vi "Get GPS Data.vi"(8 "error in (no error)":errorcluster, 10 "sensor data":string, 11 "previous partial sentence":string) -> (0 "error out":errorcluster, 2 "GPS data":T1 {"oldest read timestamp" format="%^<%.3X\n%x>T"}, 3 "remaining partial sentence":string)   [LabVIEW 2017, in "NMEA API.lvlib"]
doc: "Parses <B>sensor data</B> in the NMEA format from GPS receivers and returns common <B>GPS data</B>, such as the latitude and longitude of a reading."
uses:
  <vilib>/robotics/Protocols/NMEA/NMEA API.lvlib
  <vilib>/robotics/Protocols/NMEA/Advanced/Instrument Specific Poly VIs/GPS/Parse GLL Sentence.vi
  <vilib>/robotics/Protocols/NMEA/Advanced/Instrument Specific Poly VIs/GPS/Parse GGA Sentence.vi
  <vilib>/robotics/Protocols/NMEA/Advanced/Instrument Specific Poly VIs/GPS/Parse RMC Sentence.vi
  <vilib>/robotics/Utilities/NI_Robotics Utilities.lvlib
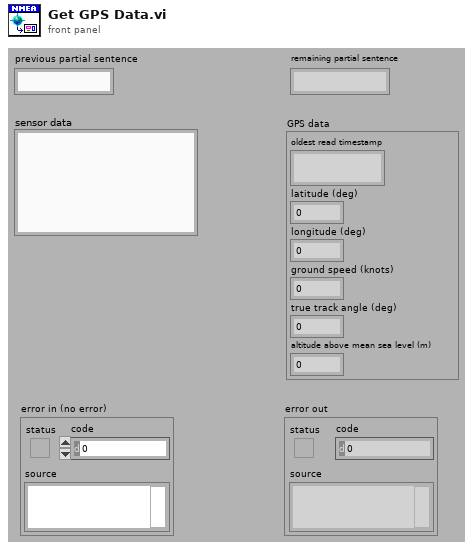
[diagram p1: front panel]
types:
  T1 = cluster{"oldest read timestamp":timestamp, "latitude (deg)":dbl, "longitude (deg)":dbl, "ground speed (knots)":dbl, "true track angle (deg)":dbl, "altitude above mean sea level (m)":dbl}
  T2 = cluster{"oldest read timestamp":timestamp, "latitude":dbl, "longitude":dbl, "speed over ground (knots)":dbl, "true track angle (deg)":dbl, "altitude above mean sea level":dbl}
  T3 = cluster{"Oldest Read Timestamp":timestamp, "Latitude":dbl, "Longitude":dbl, "Speed over Ground (Knots)":dbl, "True Track Angle (Deg)":dbl, "Altitude Above Mean Sea Level":dbl}
  T4 = typedef "NMEA API.lvlib/RMC Data.ctl" = cluster{"time of fix":cluster{"included?":bool, "time (UTC)":timestamp}, "status":cluster{"included?":bool, "value":u16}, "latitude":cluster{"included?":bool, "latitude (deg)":dbl}, "longitude":cluster{"included?":bool, "longitude (deg)":dbl}, "ground speed":cluster{"included?":bool, "speed (knots)":dbl}, "true track angle":cluster{"included?":bool, "angle (deg)":dbl}, "magnetic variation":cluster{"included?":bool, "variation (deg)":dbl}, "type of fix":cluster{"included?":bool, "mode":u16}}
  T5 = typedef "NMEA API.lvlib/GGA Data.ctl" = cluster{"time of fix":cluster{"included?":bool, "time (UTC)":timestamp}, "latitude":cluster{"included?":bool, "latitude (deg)":dbl}, "longitude":cluster{"included?":bool, "longitude (deg)":dbl}, "fix quality":cluster{"included?":bool, "quality":u16}, "number of satellites in view":cluster{"included?":bool, "number of satellites":i8}, "horizontal dilution of precision":cluster{"included?":bool, "horizontal DOP":dbl}, "altitude above mean sea level":cluster{"included?":bool, "altitude (m)":dbl}, "height of geoid above WGS84":cluster{"included?":bool, "height of geoid (m)":dbl}, "time since last DGPS update":cluster{"included?":bool, "time (s)":dbl}, "DGPS station ID number":cluster{"included?":bool, "station ID number":dbl}}
  T6 = typedef "NMEA API.lvlib/GLL Data.ctl" = cluster{"latitude":cluster{"included?":bool, "latitude (deg)":dbl}, "longitude":cluster{"included?":bool, "longitude (deg)":dbl}, "time of fix":cluster{"included?":bool, "time (UTC)":timestamp}, "status":cluster{"included?":bool, "value":u16}, "type of fix":cluster{"included?":bool, "mode":u16}}
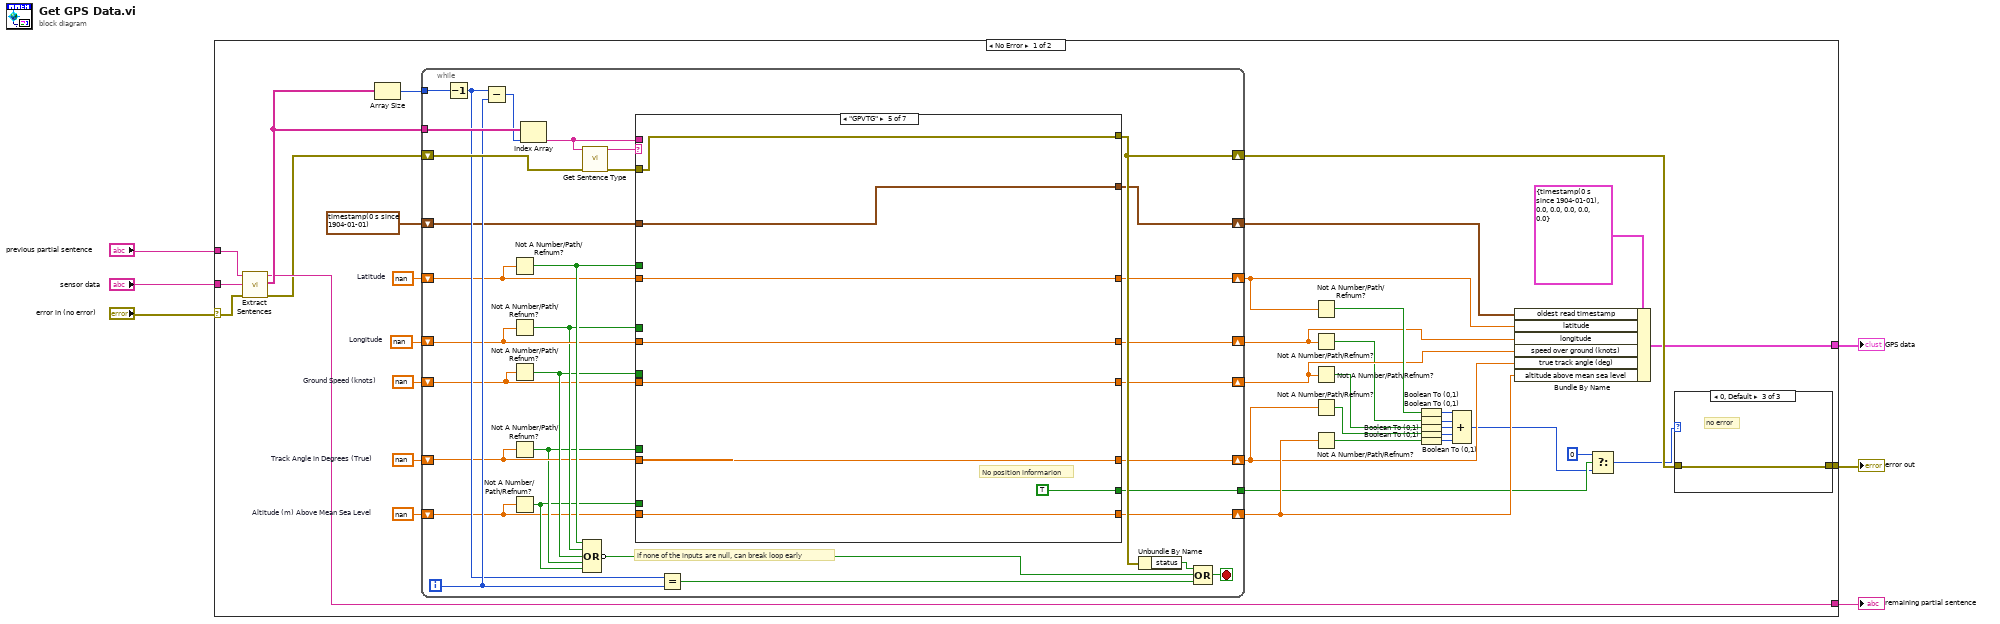
[diagram p0: block diagram]
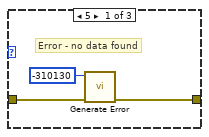
[diagram p2: hidden frame]
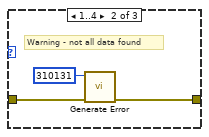
[diagram p3: hidden frame]
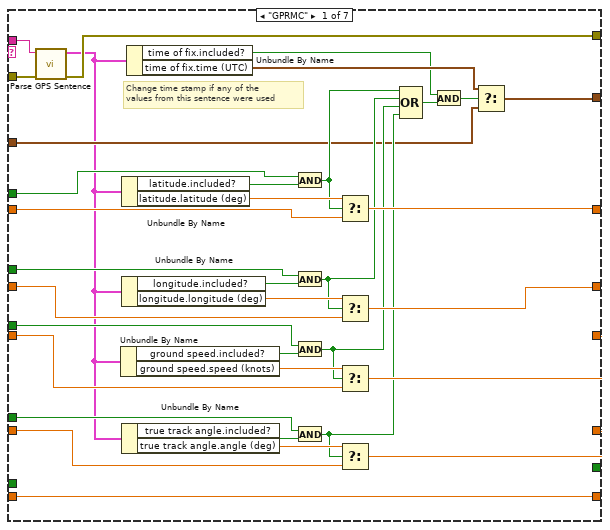
[diagram p4: hidden frame]
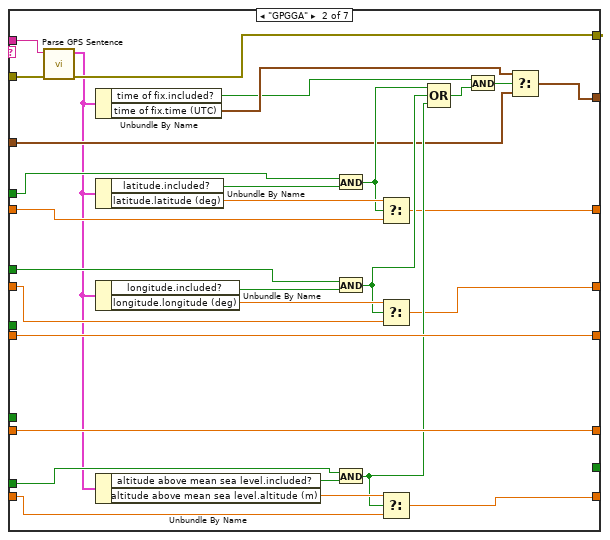
[diagram p5: hidden frame]
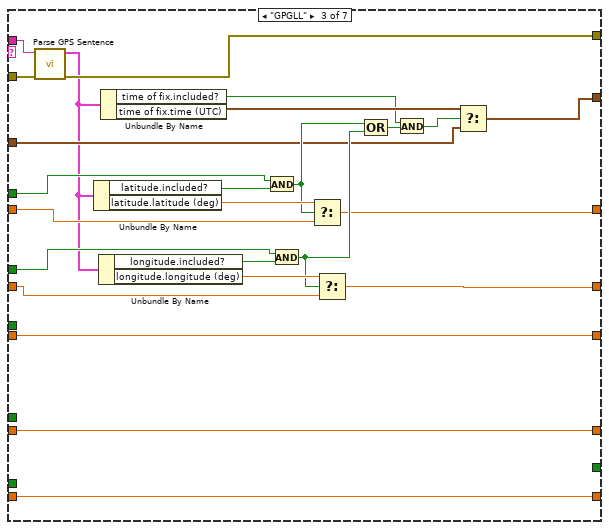
[diagram p6: hidden frame]
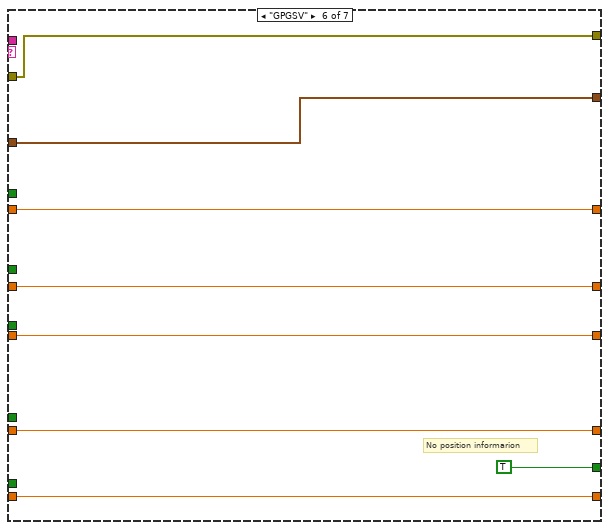
[diagram p8: hidden frame]
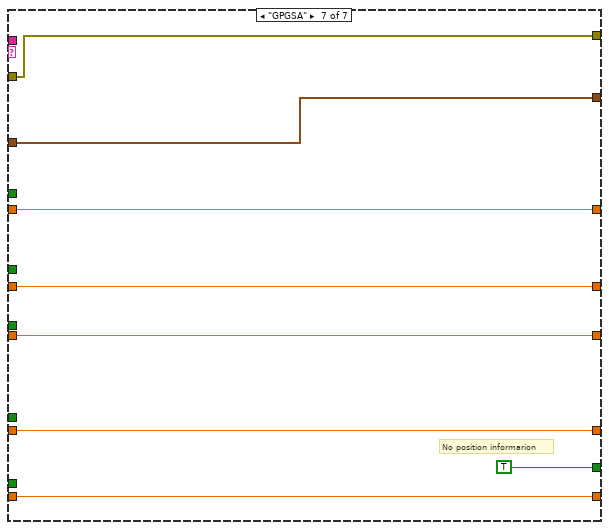
[diagram p9: hidden frame]
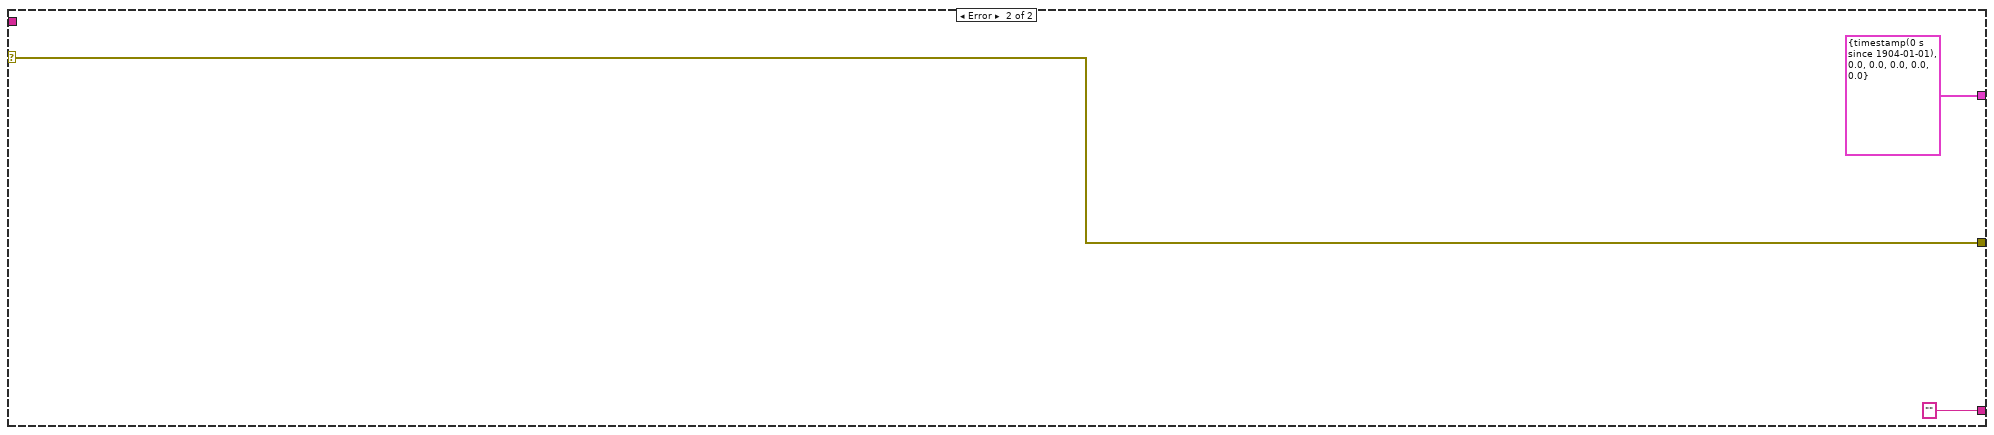
[diagram p10: hidden frame]
diagram:
  n1 = case shown="No Error" "error in (no error)" {
    selector: "error in (no error)" -> [w21 w206]
    tunnel: [w41 w206] -> w5
    tunnel: "sensor data" -> [w30 _]
    tunnel: "previous partial sentence" -> [w29 _]
    tunnel: [w28 T3 {"Oldest Read Timestamp"=timestamp(0 s since 1904-01-01), "Latitude"=0.0, "Longitude"=0.0, "Speed over Ground (Knots)"=0.0, "True Track Angle (Deg)"=0.0, "Altitude Above Mean Sea Level"=0.0} ("GPS Data")] -> w2
    tunnel: [w22 "" ("After Last Sentence")] -> w1
    frame No Error {
      w34 = nan  # Altitude (m) Above Mean Sea Level
      w35 = nan  # Track Angle in Degrees (True)
      w32 = nan  # Ground Speed (knots)
      w36 = nan  # Longitude
      w37 = nan  # Latitude
      n2 = call <vilib>:"Extract Sentences.vi"("error in (no error)"=w21, "sensor data"=w30, "previous partial sentence"=w29) -> ("error out"=w20:errorcluster, "complete sentences"=w40:string[], "remaining partial sentence"=w22:string)  [unwired: 4 in, 2 out]
      n3 = Array Size(array=w40) -> (size(s)=w39:i32)
      n4 = while {
        tunnel: w40 -> [w81]
        shift-right: [w77] -> w42
        shift-left: w20 -> [w79]
        shift-right: [w71] -> w43
        shift-left: timestamp(0 s since 1904-01-01) ("Time of Fix (UTC)") -> [w64]
        shift-right: [w69] -> w31
        shift-left: w37 -> [w62]
        shift-right: [w68] -> w15
        shift-left: w36 -> [w61]
        shift-right: [w76] -> w17
        shift-left: w35 -> [w57]
        shift-right: [w70] -> w18
        shift-left: w34 -> [w54]
        tunnel: w39 -> [w66]
        shift-right: [w67] -> w16
        shift-left: w32 -> [w58]
        tunnel: [w51] -> w10
        i -> [w74]
        stop <- w82 stop-if-true
        # "if none of the inputs are null, can break loop early"
        n5 = Decrement(x=w66) -> (x-1=w65:i32)
        n6 = Subtract(x=w65, y=w74) -> (x-y=w75:i32)
        n7 = Not A Number/Path/Refnum?(number/path/refnum=w62) -> (NaN/Path/Refnum?=w63:bool)
        n8 = Not A Number/Path/Refnum?(number/path/refnum=w61) -> (NaN/Path/Refnum?=w60:bool)
        n9 = Not A Number/Path/Refnum?(number/path/refnum=w58) -> (NaN/Path/Refnum?=w59:bool)
        n10 = Not A Number/Path/Refnum?(number/path/refnum=w57) -> (NaN/Path/Refnum?=w56:bool)
        n11 = Not A Number/Path/Refnum?(number/path/refnum=w54) -> (NaN/Path/Refnum?=w55:bool)
        n12 = Index Array(array=w81, index=w75) -> (element=w53:string)
        n13 = call <vilib>:"Get Sentence Type.vi"("error in (no error)"=w79, "sentence"=w53) -> ("error out"=w78:errorcluster, "sentence type"=w52:string)  [unwired: 1 in, 7 out]
        n14 = Compound Arithmetic op=OR(w63, w60, w59, w56, w55) -> (invert w72:bool)
        n15 = case shown="\"GPVTG\"" w52 {
          tunnel: w78 -> [w117 w147 w172 w179 w187 w195 w203]
          tunnel: [w116 w145 w170 w179 w187 w195 w203] -> w77
          tunnel: [w110 w146 w171 w178 w186 w194 w202] -> w76
          tunnel: w53 -> [w84 w119 w149 _ _ _ _]
          tunnel: w64 -> [w89 w122 w151 w177 w185 w193 w201]
          tunnel: w62 -> [w96 w127 w158 w175 w183 w191 w199]
          tunnel: w61 -> [w101 w133 w164 w174 w182 w190 w198]
          tunnel: w57 -> [w111 w146 w171 w178 w186 w194 w202]
          tunnel: w54 -> [w115 w141 w169 w176 w184 w192 w200]
          tunnel: w63 -> [w98 w128 w159 _ _ _ _]
          tunnel: w60 -> [w103 w135 w160 _ _ _ _]
          tunnel: w59 -> [w105 _ _ _ _ _ _]
          tunnel: w56 -> [w113 _ _ _ _ _ _]
          tunnel: w55 -> [_ w140 _ _ _ _ _]
          tunnel: [w85 w121 w150 w177 w185 w193 w201] -> w71
          tunnel: [w115 w138 w169 w176 w184 w192 w200] -> w70
          tunnel: [w95 w129 w157 w175 w183 w191 w199] -> w69
          tunnel: [w106 w144 w168 w173 w181 w189 w197] -> w67
          tunnel: [w100 w132 w163 w174 w182 w190 w198] -> w68
          tunnel: w58 -> [w107 w144 w168 w173 w181 w189 w197]
          tunnel: [_ _ _ _ TRUE TRUE TRUE] -> w51
          frame "GPRMC" {
            # "Change time stamp if any of the\nvalues from this sentence were used"
            n16 = call-poly <vilib>:"Parse GPS Sentence.vi"("error in (no error)"=w117, "RMC sentence"=w84) -> ("error out"=w116:errorcluster, "RMC data"=w83:T4)  [unwired: 1 in, 7 out]
            n17 = Unbundle By Name(w83) -> ("ground speed.included?"=w109:bool, "ground speed.speed (knots)"=w108:dbl)
            n18 = Unbundle By Name(w83) -> ("latitude.included?"=w99:bool, "latitude.latitude (deg)"=w97:dbl)
            n19 = Unbundle By Name(w83) -> ("longitude.included?"=w104:bool, "longitude.longitude (deg)"=w102:dbl)
            n20 = Unbundle By Name(w83) -> ("true track angle.included?"=w114:bool, "true track angle.angle (deg)"=w112:dbl)
            n21 = Unbundle By Name(w83) -> ("time of fix.included?"=w87:bool, "time of fix.time (UTC)"=w88:timestamp)
            n22 = And(x=w98, y=w99) -> (x .and. y?=w94:bool)
            n23 = And(x=w103, y=w104) -> (x .and. y?=w93:bool)
            n24 = And(x=w105, y=w109) -> (x .and. y?=w92:bool)
            n25 = And(x=w113, y=w114) -> (x .and. y?=w91:bool)
            n26 = Select(t=w97, s=w94, f=w96) -> (s? t:f=w95:dbl)
            n27 = Select(t=w102, s=w93, f=w101) -> (s? t:f=w100:dbl)
            n28 = Select(t=w108, s=w92, f=w107) -> (s? t:f=w106:dbl)
            n29 = Select(t=w112, s=w91, f=w111) -> (s? t:f=w110:dbl)
            n30 = Compound Arithmetic op=OR(w94, w93, w92, w91) -> (w90:bool)
            n31 = And(x=w87, y=w90) -> (x .and. y?=w86:bool)
            n32 = Select(t=w88, s=w86, f=w89) -> (s? t:f=w85:timestamp)
          }
          frame "GPGGA" {
            n33 = call-poly <vilib>:"Parse GPS Sentence.vi"("error in (no error)"=w147, "GGA sentence"=w119) -> ("error out"=w145:errorcluster, "GGA data"=w118:T5)  [unwired: 1 in, 7 out]
            n34 = Unbundle By Name(w118) -> ("time of fix.included?"=w124:bool, "time of fix.time (UTC)"=w125:timestamp)
            n35 = Unbundle By Name(w118) -> ("latitude.included?"=w131:bool, "latitude.latitude (deg)"=w130:dbl)
            n36 = Unbundle By Name(w118) -> ("longitude.included?"=w137:bool, "longitude.longitude (deg)"=w136:dbl)
            n37 = Unbundle By Name(w118) -> ("altitude above mean sea level.included?"=w143:bool, "altitude above mean sea level.altitude (m)"=w142:dbl)
            n38 = And(x=w128, y=w131) -> (x .and. y?=w126:bool)
            n39 = And(x=w135, y=w137) -> (x .and. y?=w134:bool)
            n40 = And(x=w140, y=w143) -> (x .and. y?=w139:bool)
            n41 = Select(t=w130, s=w126, f=w127) -> (s? t:f=w129:dbl)
            n42 = Select(t=w136, s=w134, f=w133) -> (s? t:f=w132:dbl)
            n43 = Select(t=w142, s=w139, f=w141) -> (s? t:f=w138:dbl)
            n44 = Compound Arithmetic op=OR(w126, w134, w139) -> (w120:bool)
            n45 = And(x=w124, y=w120) -> (x .and. y?=w123:bool)
            n46 = Select(t=w125, s=w123, f=w122) -> (s? t:f=w121:timestamp)
          }
          frame "GPGLL" {
            n47 = call-poly <vilib>:"Parse GPS Sentence.vi"("error in (no error)"=w172, "GLL sentence"=w149) -> ("error out"=w170:errorcluster, "GLL data"=w148:T6)  [unwired: 2 in, 6 out]
            n48 = Unbundle By Name(w148) -> ("latitude.included?"=w162:bool, "latitude.latitude (deg)"=w161:dbl)
            n49 = Unbundle By Name(w148) -> ("longitude.included?"=w167:bool, "longitude.longitude (deg)"=w166:dbl)
            n50 = Unbundle By Name(w148) -> ("time of fix.included?"=w154:bool, "time of fix.time (UTC)"=w155:timestamp)
            n51 = And(x=w159, y=w162) -> (x .and. y?=w156:bool)
            n52 = And(x=w160, y=w167) -> (x .and. y?=w165:bool)
            n53 = Select(t=w161, s=w156, f=w158) -> (s? t:f=w157:dbl)
            n54 = Select(t=w166, s=w165, f=w164) -> (s? t:f=w163:dbl)
            n55 = Compound Arithmetic op=OR(w156, w165) -> (w152:bool)
            n56 = And(x=w154, y=w152) -> (x .and. y?=w153:bool)
            n57 = Select(t=w155, s=w153, f=w151) -> (s? t:f=w150:timestamp)
          }
          frame "", Default {
          }
          frame "GPVTG" {
            # "No position informarion"
          }
          frame "GPGSV" {
            # "No position informarion"
          }
          frame "GPGSA" {
            # "No position informarion"
          }
        }
        n58 = Equal?(x=w65, y=w74) -> (x = y?=w80:bool)
        n59 = Unbundle By Name(w77) -> ("status"=w73:bool)
        n60 = Compound Arithmetic op=OR(w73, w72, w80) -> (w82:bool)
      }
      n61 = Not A Number/Path/Refnum?(number/path/refnum=w31) -> (NaN/Path/Refnum?=w19:bool)
      n62 = Not A Number/Path/Refnum?(number/path/refnum=w15) -> (NaN/Path/Refnum?=w14:bool)
      n63 = Not A Number/Path/Refnum?(number/path/refnum=w16) -> (NaN/Path/Refnum?=w13:bool)
      n64 = Not A Number/Path/Refnum?(number/path/refnum=w17) -> (NaN/Path/Refnum?=w12:bool)
      n65 = Not A Number/Path/Refnum?(number/path/refnum=w18) -> (NaN/Path/Refnum?=w11:bool)
      n66 = Boolean To (0,1)(Boolean=w19) -> (0, 1=w27:i16)
      n67 = Boolean To (0,1)(Boolean=w14) -> (0, 1=w26:i16)
      n68 = Boolean To (0,1)(Boolean=w13) -> (0, 1=w25:i16)
      n69 = Boolean To (0,1)(Boolean=w12) -> (0, 1=w24:i16)
      n70 = Boolean To (0,1)(Boolean=w11) -> (0, 1=w23:i16)
      n71 = Compound Arithmetic op=ADD(w27, w26, w25, w24, w23) -> (w9:i16)
      n72 = Bundle By Name(cluster=T2 {"oldest read timestamp"=timestamp(0 s since 1904-01-01), "latitude"=0.0, "longitude"=0.0, "speed over ground (knots)"=0.0, "true track angle (deg)"=0.0, "altitude above mean sea level"=0.0} ("GPS Data"), "oldest read timestamp"=w43, "latitude"=w31, "longitude"=w15, "speed over ground (knots)"=w16, "true track angle (deg)"=w17, "altitude above mean sea level"=w18) -> (w28:T2)
      n73 = Select(t=i16 0, s=w10, f=w9) -> (s? t:f=w8:i16)
      n74 = case shown="0, Default" w8 {
        tunnel: w42 -> [w46 w48 w50]
        tunnel: [w45 w47 w50] -> w41
        frame 5 {
          # "Error - no data found"
          n75 = call <vilib>:"Generate Error.vi"("error in (no error)"=w46, "code"=-310130) -> ("error out"=w45:errorcluster)  [unwired: 9 in]
        }
        frame 1..4 {
          # "Warning - not all data found"
          n76 = call <vilib>:"Generate Error.vi"("error in (no error)"=w48, "code"=310131) -> ("error out"=w47:errorcluster)  [unwired: 9 in]
        }
        frame 0, Default {
          # "no error"
        }
      }
    }
    frame Error {
    }
  }
  "error out" <- w5
  "remaining partial sentence" <- w1
  "GPS data" <- w2
